vi "SetBinning.vi"(8 "error in (no error)":errorcluster, 9 "Setting.Binning.BinY":i32, 10 "Setting.Binning.BinX":i32, 11 "Camera_Prime95B in":refnum<class "Camera_Prime95B.lvclass">) -> (0 "error out":errorcluster, 3 "Camera_Prime95B out":refnum<class "Camera_Prime95B.lvclass">)   [LabVIEW 2020, in "Camera_Prime95B.lvlib" / "Camera_Prime95B.lvclass"]
uses:
  Camera_Prime95B.lvclass
  Camera_Prime95B.lvclass/Camera_Prime95B.ctl
  E:/Development/DevHardSoftware/MicroscopyFramework/Model/Hardware Layer/Real Hardware/Camera_Prime95B/Camera_Prime95B/Dependencies/PVCamNET.dll
  Dependencies/PVCamNET.dll
  Controls/Wait For Stop Status.ctl
  Hardware Abstraction Layer/Component/Camera/Camera/Camera.lvclass
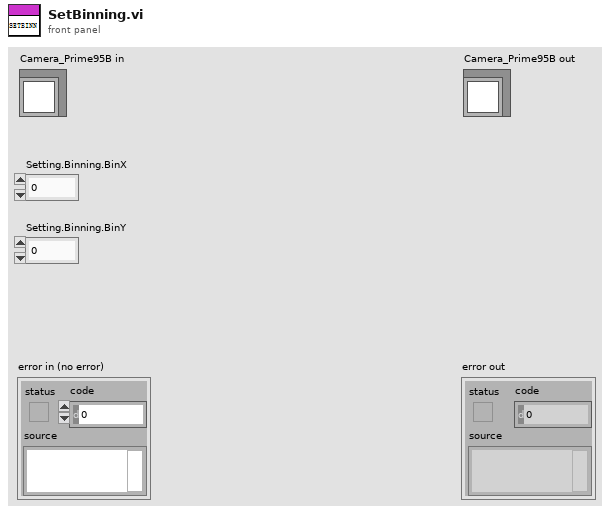
[diagram p1: front panel]
types:
  T1 = typedef "Device.lvlib/DeviceStatus.ctl" = i32
  T2 = typedef "Camera_Prime95B.lvlib/Camera_Prime95B.lvclass/Wait For Stop Status.ctl" = i32
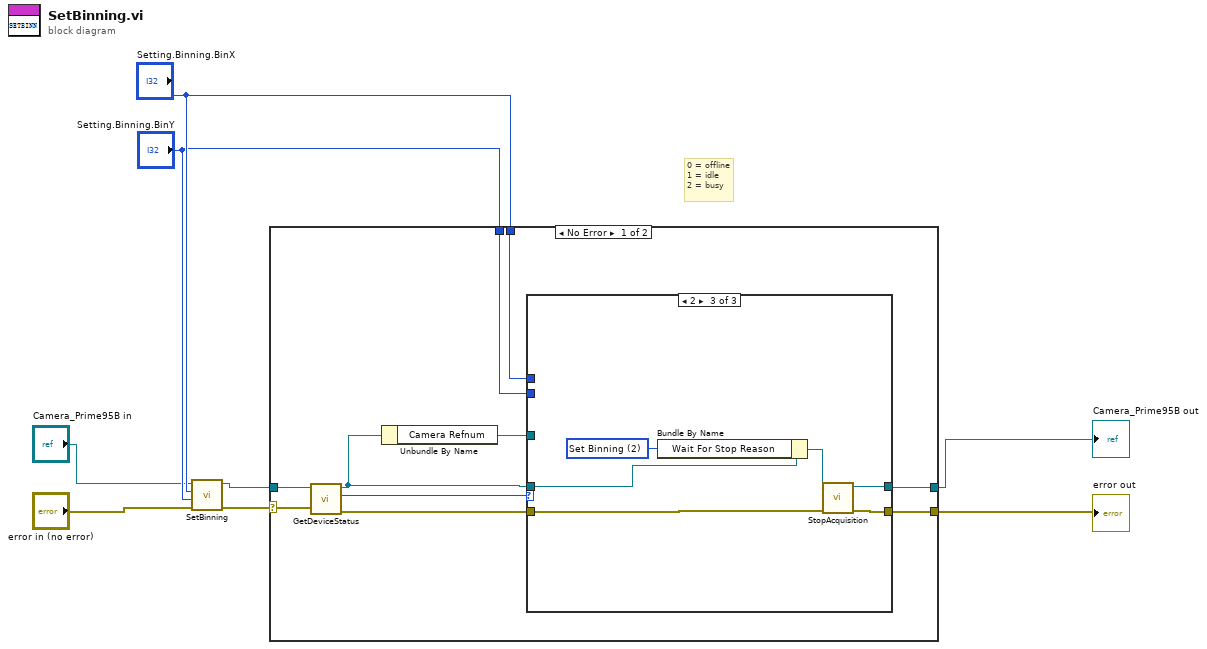
[diagram p0: block diagram]
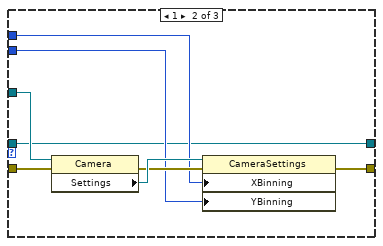
[diagram p3: hidden frame]
diagram:
  # "0 = offline\n1 = idle\n2 = busy"
  n1 = call-parent "SetBinning.vi"("error in (no error)"="error in (no error)", "Setting.Binning.BinY"="Setting.Binning.BinY", "Setting.Binning.BinX"="Setting.Binning.BinX", "Camera in"="Camera_Prime95B in") -> ("error out"=w6:errorcluster, "Camera out"=w3:refnum<class "Camera_Prime95B.lvclass">)  [unwired: 6 in]
  n2 = case shown="No Error" w6 {
    selector: w6 -> [w15 w36]
    tunnel: [w16 w36] -> w1
    tunnel: "Setting.Binning.BinX" -> [w18 _]
    tunnel: "Setting.Binning.BinY" -> [w17 _]
    tunnel: [w10 w35] -> w2
    tunnel: w3 -> [w9 w35]
    frame No Error {
      n3 = call-dynamic "GetDeviceStatus.vi"("error in (no error)"=w15, "Camera_Prime95B in"=w9) -> ("error out"=w13:errorcluster, "Status"=w14:T1, "Camera_Prime95B out"=w11:refnum<class "Camera_Prime95B.lvclass">)  [unwired: 7 in]
      n4 = Unbundle By Name(w11) -> ("Camera Refnum"=w12:refnum<k24>)
      n5 = case shown="2" w14 {
        tunnel: [w19 w28 w33] -> w16
        tunnel: w12 -> [_ w25 _]
        tunnel: w18 -> [_ w24 _]
        tunnel: w17 -> [_ w23 _]
        tunnel: w13 -> [w19 w22 w34]
        tunnel: w11 -> [w20 w21 w30]
        tunnel: [w20 w21 w31] -> w10
        frame 0, Default {
        }
        frame 1 {
          n6 = property class="Camera"(reference=w25, error in=w22) -> (error out=w26:errorcluster, "Settings"=w27:refnum<k24>)  [unwired: 1 out]
          n7 = property class="CameraSettings"(reference=w27, error in=w26, "XBinning"=w24, "YBinning"=w23) -> (error out=w28:errorcluster)  [unwired: 1 out]
        }
        frame 2 {
          w32 = T2 2 items=["None", "Set Exposure", "Set Binning", "Set ROI", "Senquen Acq", ""] ("Wait For Stop Reason")
          n8 = Bundle By Name(cluster=w30, "Wait For Stop Reason"=w32) -> (w29:refnum<class "Camera_Prime95B.lvclass">)
          n9 = call-dynamic "StopAcquisition.vi"("error in (no error)"=w34, "Camera_Prime95B in"=w29) -> ("error out"=w33:errorcluster, "Camera_Prime95B out"=w31:refnum<class "Camera_Prime95B.lvclass">)  [unwired: 8 in]
        }
      }
    }
    frame Error {
    }
  }
  "error out" <- w1
  "Camera_Prime95B out" <- w2
